vi "测试-灰度变换BCG Lookup.vi"() -> ()   [LabVIEW 2018]
doc: "This example shows how to apply a brightness, contrast, and gamma correction lookup table to an image. These transformations are usually applied to an image to improve its quality as required by a particular application."
uses:
  <vilib>/vision/NI_Vision_Development_Module.lvlib
panel:
  out "Hist-Src":T1(graph)
  out "Image Source":T2(plugin-control)
  out "Dst":T2(plugin-control) caption="Lut Image"
  out "Hist-Dst":T1(graph)
  in  "Stop Button":bool
  in  "BCG":T3={"Brightness"=171.0, "Contrast"=56.0, "Gamma"=2.0} {"Gamma" min=0.1 max=10 step=0.01 scale=10.0..0.1; "Contrast" min=1 max=89 step=1 scale=30.0..60.0; "Brightness" min=0 max=255 step=1 scale=0.0..255.0}
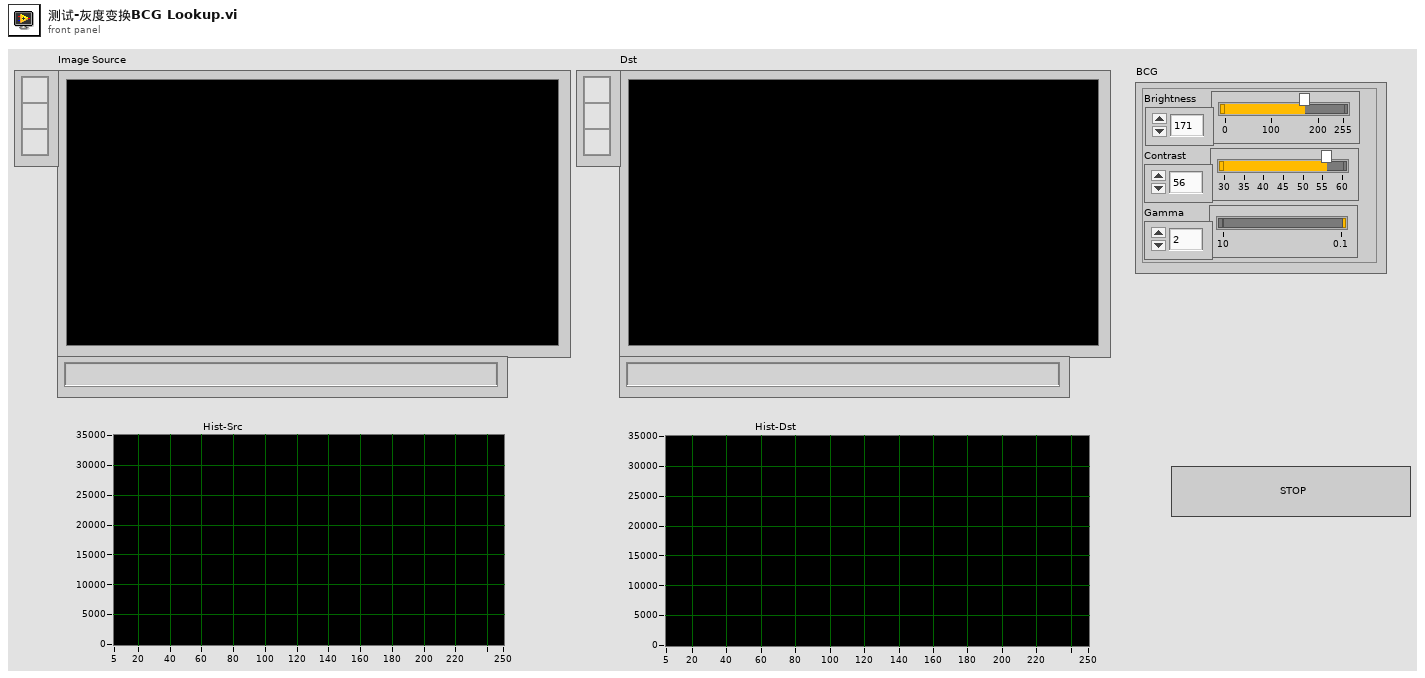
[diagram p1: front panel]
types:
  T1 = cluster{"Starting Value":sgl, "Incremental Value":sgl, "Histogram":u32[]}
  T2 = typedef "IMAQ Image.ctl" = refnum<image>
  T3 = cluster{"Brightness":sgl, "Contrast":sgl, "Gamma":sgl}
  T4 = typedef "Image Type" = u32
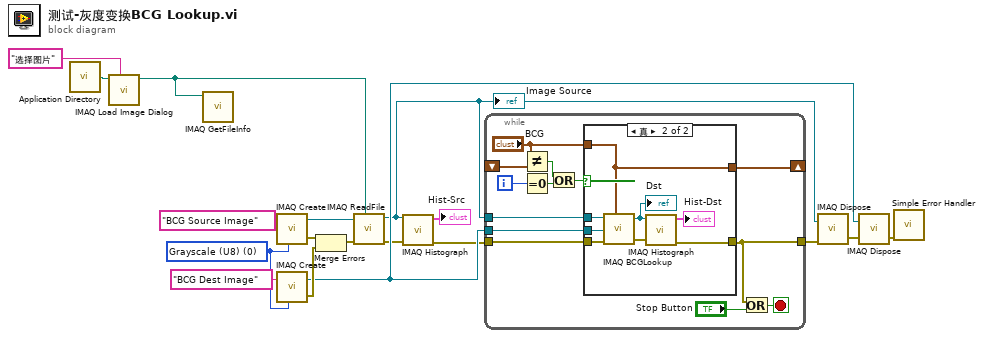
[diagram p0: block diagram]
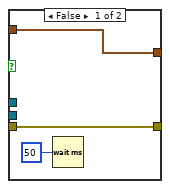
[diagram p2: hidden frame]
diagram:
  w9 = T4 0 items=["Grayscale (U8)", "Grayscale (I16)", "Grayscale (SGL)", "Complex (CSG)", "RGB (U32)", "HSL (U32)", "RGB (U64)", "Grayscale (U16)"] ("Image Type")
  n1 = call <vilib>:"Application Directory.vi"() -> ("Application Directory"=w3:path)
  n2 = call "IMAQ Load Image Dialog"("Prompt"="选择图片" ("prompt"), "Start Path"=w3) -> ("Path"=w1:path)  [unwired: 7 in, 2 out]
  n3 = call "IMAQ GetFileInfo"("File Path"=w1) -> ()  [unwired: 4 in, 7 out]
  n4 = call "IMAQ Create"("Image Name"="BCG Source Image", "Image Type"=w9) -> ("New Image"=w16:T2, "error out"=w15:errorcluster)  [unwired: 3 in]
  n5 = call "IMAQ Create"("Image Name"="BCG Dest Image", "Image Type"=w9) -> ("New Image"=w10:T2, "error out"=w14:errorcluster)  [unwired: 3 in]
  n6 = Merge Errors(w15, w14) -> (w13:errorcluster)
  n7 = call "IMAQ ReadFile"("File Path"=w1, "error in (no error)"=w13, "Image"=w16) -> ("error out"=w7:errorcluster, "Image Out"=w6:T2)  [unwired: 4 in, 3 out]
  "Image Source" <- w6
  n8 = call "IMAQ Histograph"("error in (no error)"=w7, "Image"=w6) -> ("error out"=w5:errorcluster, "Histogram Graph"=→"Hist-Src":T1)  [unwired: 6 in, 2 out]
  n9 = while {
    tunnel: w5 -> [w31]
    tunnel: w6 -> [w30]
    tunnel: w10 -> [w29]
    shift-right: [w28] -> _
    shift-left: _ -> [w27]
    tunnel: [w20] -> w18
    i -> [w25]
    stop <- w19 stop-if-true
    n10 = Not Equal?(x="BCG", y=w27) -> (x != y?=w24:bool)
    n11 = Equal To 0?(x=w25) -> (x = 0?=w23:bool)
    n12 = Or(x=w24, y=w23) -> (x .or. y?=w22:bool)
    n13 = case shown="真" w22 {
      tunnel: w31 -> [w34 w42]
      tunnel: w30 -> [_ w41]
      tunnel: "BCG" -> [w33 w39]
      tunnel: w29 -> [_ w40]
      tunnel: [w33 w39] -> w28
      tunnel: [w34 w37] -> w20
      frame False {
        n14 = Wait (ms)(milliseconds to wait=u32 50) -> ()  [unwired: 1 out]
      }
      frame True {
        n15 = call "IMAQ BCGLookup"("Image Src"=w41, "BCG Values"=w39, "Image Dst"=w40, "error in (no error)"=w42) -> ("Image Dst Out"=w35:T2, "error out"=w38:errorcluster)  [unwired: 3 in]
        "Dst" <- w35
        n16 = call "IMAQ Histograph"("error in (no error)"=w38, "Image"=w35) -> ("error out"=w37:errorcluster, "Histogram Graph"=→"Hist-Dst":T1)  [unwired: 6 in, 2 out]
      }
    }
    n17 = Or(x=w20, y="Stop Button") -> (x .or. y?=w19:bool)
  }
  n18 = call "IMAQ Dispose"("Image"=w6, "error in (no error)"=w18) -> ("error out"=w11:errorcluster)  [unwired: 4 in]
  n19 = call "IMAQ Dispose"("Image"=w10, "error in (no error)"=w11) -> ("error out"=w12:errorcluster)  [unwired: 4 in]
  n20 = call <vilib>:"Simple Error Handler.vi"("error in (no error)"=w12) -> ()  [unwired: 4 in, 5 out]
